vi "Config Mismatch Alert UI.vi"(11 "System Config Module in":refnum<class "System Config Module.lvclass">) -> ()   [LabVIEW 2020, in "Volatus.lvlib" / "System Config Module.lvclass"]
uses:
  System Config Module.lvclass
panel:
  in  "Config Hash":string
  in  "Config Version":string
  out "Message":string="Configuration mismatch was detected. The program will likely have improper functionality unless all configurations match."
  in  "Array":T1(array[cluster])
  # "This Node"
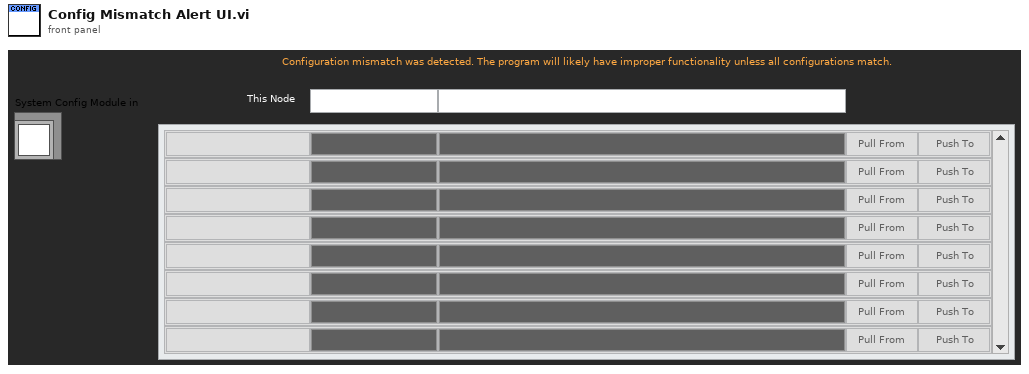
[diagram p1: front panel]
types:
  T1 = cluster{"Node":string, "Config Version":string, "Config Hash":string, "Pull":bool, "Push":bool, "Version Color":u32, "Hash Color":u32}[]
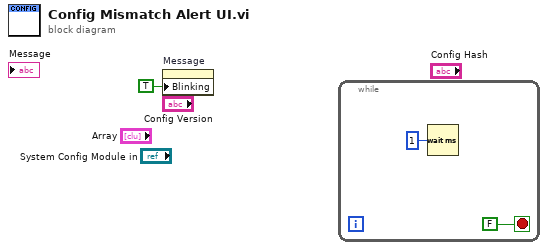
[diagram p0: block diagram]
diagram:
  n1 = property on="Message" class="Str"("Blinking"=TRUE) -> ()  [unwired: 2 in, 2 out]
  n2 = while {
    stop <- FALSE stop-if-true
    n3 = Wait (ms)(milliseconds to wait=u32 1) -> ()  [unwired: 1 out]
  }
